vi "Performance Monitor.vi"(8 "error in (no error)":errorcluster) -> ()   [LabVIEW 2011]
uses:
  Shared/cRIO Performance Details.ctl
  Robot Global Data.vi
  <vilib>/NI_Real-Time Target Support.lvlib
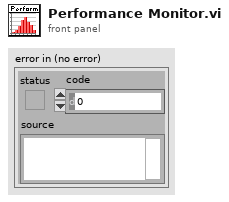
[diagram p1: front panel]
types:
  T1 = typedef "cRIO Performance Details.ctl" = cluster{"CPU Utilization":dbl, "RAM total (bytes)":u32, "RAM available (bytes)":u32, "Flash size (bytes)":i64, "Flash free (bytes)":i64}
  T2 = typedef "NI_Real-Time Target Support.lvlib/RT CPU Load.ctl" = cluster{"Total (%)":dbl, "Time Critical (%)":dbl, "Timed Structures (%)":dbl, "High (%)":dbl, "Above Normal (%)":dbl, "Normal (%)":dbl, "Background (%)":dbl, "Idle (%)":dbl, "ISR (%)":dbl}
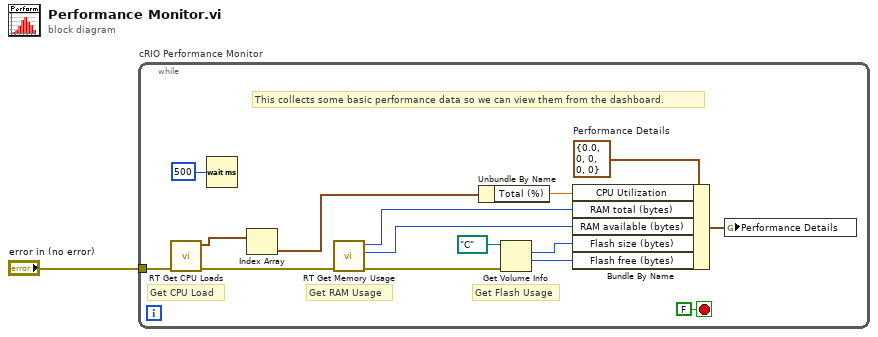
[diagram p0: block diagram]
diagram:
  n1 = while "cRIO Performance Monitor" {
    tunnel: "error in (no error)" -> [w5]
    stop <- FALSE stop-if-true
    w6 = T1 {"CPU Utilization"=0.0, "RAM total (bytes)"=0, "RAM available (bytes)"=0, "Flash size (bytes)"=0, "Flash free (bytes)"=0}  # Performance Details
    # "This collects some basic performance data so we can view them from the dashboard."
    # "Get Flash Usage"
    # "Get RAM Usage"
    # "Get CPU Load"
    n2 = call <vilib>:"RT Get CPU Loads.vi"("error in (no error)"=w5) -> ("error out"=w16:errorcluster, "CPU loads"=w4:T2[])  [unwired: 9 in]
    n3 = Wait (ms)(milliseconds to wait=u32 500) -> ()  [unwired: 1 out]
    n4 = Index Array(array=w4) -> (element=w3:T2)  [unwired: 1 in]
    n5 = call <vilib>:"RT Get Memory Usage.vi"("error in (no error)"=w16) -> ("error out"=w13:errorcluster, "available (bytes)"=w9:u32, "total (bytes)"=w8:u32)  [unwired: 7 in, 1 out]
    n6 = Unbundle By Name(w3) -> ("Total (%)"=w2:dbl)
    n7 = Get Volume Info(8:w13, 11:path "C:/" ("path")) -> (1:w10:i64, 2:w11:i64)  [unwired: 4 out]
    n8 = Bundle By Name(cluster=w6, "CPU Utilization"=w2, "RAM total (bytes)"=w8, "RAM available (bytes)"=w9, "Flash size (bytes)"=w11, "Flash free (bytes)"=w10) -> (w7:T1)
    n9 = global write "Robot Global Data.vi" "Performance Details"(w7) -> ()
  }
